vi "Main Tclk.vi"() -> ()   [LabVIEW 2018] (continued)
                        n671 = local read "Email recipents file"() -> (w5881:path)
                        n672 = Open/Create/Replace File(file path (use dialog)=w5881, operation (0:open)=T49."replace or create") -> (refnum out=w5882:refnum<file>, error out=w5883:errorcluster)  [unwired: 4 in, 1 out]
                        n673 = Write to Text File(file (use dialog)=w5882, text=w5884, error in=w5883) -> (refnum out=w5885:refnum<file>, error out=w5886:errorcluster)  [unwired: 1 in, 1 out]
                        n674 = Close File(refnum=w5885, error in=w5886) -> ()  [unwired: 2 out]
                      }
                      frame #4 {
                        n675 = local read "Hardware Configuration"() -> (w5948:T25)
                        n676 = local read "SEM Scan Parameters"() -> (w5932:T26)
                        n677 = local read "SEM Options"() -> (w5949:T27)
                        n678 = local read "SEM Status"() -> (w5950:T12)
                        n679 = local read "X full scale (V)"() -> (w5951:sgl)
                        n680 = local read "Mid Mag SEM"() -> (w5947:T29)
                        n681 = local read "SEM Mid Mag Scan Parameters"() -> (w5946:T5)
                        n682 = Unbundle By Name(w5947) -> ("X size (um)"=w5943:sgl, "Y size (um)"=w5942:sgl, "X center (um)"=w5941:dbl, "Y center (um)"=w5940:dbl, "Mid mag scan rate (Hz)"=w5945:u32, "Pixel size (nm)"=w5944:sgl)
                        n683 = call "SEM Scan Parameter Coerce.vi"("X full scale (V)"=w5951, "AI upper limit"=50000000.0, "SEM Status"=w5950, "SEM Options"=w5949, "SEM Scan Parameters"=w5932, "Hardware Configuration"=w5948) -> ("Coerced SEM Scan Parameters"=w5952:T5, "SEM FOV"=w5931:dbl, "Detector number"=w5930:i16)  [unwired: 3 in]
                        n684 = local write "Detector number"(w5930) -> ()
                        n685 = local write "SEM FOV"(w5931) -> ()
                        n686 = Bundle By Name(cluster=w5946, "X size (um)"=w5943, "Y size (um)"=w5942, "X center (um)"=w5941, "Y center (um)"=w5940, "Scan rate (Hz)"=w5945, "Pixel size (nm)"=w5944, "X size auto"=TRUE) -> (w5939:T5)
                        n687 = call "SEM Scan Parameter Coerce.vi"("X full scale (V)"=w5951, "SEM Status"=w5950, "SEM Options"=w5949, "SEM Scan Parameters"=w5939, "Hardware Configuration"=w5948) -> ("Coerced SEM Scan Parameters"=w5953:T5)  [unwired: 4 in, 2 out]
                        n688 = Unbundle By Name(w5953) -> ("X size (um)"=w5938:sgl, "Y size (um)"=w5937:sgl, "X center (um)"=w5936:dbl, "Y center (um)"=w5935:dbl, "Scan rate (Hz)"=w5934:u32, "Pixel size (nm)"=w5933:sgl)
                        n689 = Bundle By Name(cluster=w5947, "X size (um)"=w5938, "Y size (um)"=w5937, "X center (um)"=w5936, "Y center (um)"=w5935, "Mid mag scan rate (Hz)"=w5934, "Pixel size (nm)"=w5933) -> (w5954:T29)
                        n690 = local write "SEM Scan Parameters"(w5952) -> ()
                        n691 = local write "SEM Mid Mag Scan Parameters"(w5953) -> ()
                        n692 = local write "Mid Mag SEM"(w5954) -> ()
                      }
                      frame #5 {
                        n693 = local read "Reheat from last"() -> (w5955:bool)
                        n694 = case shown="True" w5955 {
                          frame False {
                          }
                          frame True {
                            n695 = local read "SEM Scan Parameters"() -> (w5960:T26)
                            n696 = Unbundle By Name(w5960) -> ("X center (um)"=w5959:sgl, "Y center (um)"=w5958:sgl, "Y stig"=w5957:sgl[][])
                            n697 = local write "Pre-reheat X center (um)"(w5959) -> ()
                            n698 = local write "Pre-reheat Y center (um)"(w5958) -> ()
                            n699 = local write "Pre-reheat Y stig"(w5957) -> ()
                            n700 = local write "Status Tabs"(T11."Re-engage" ("Status Tabs")) -> ()
                          }
                        }
                      }
                    }
                  }
                }
              }
              frame #1 {
                n701 = local read "Machine Type"() -> (w5977:u8)
                n702 = local read "Milling para"() -> (w5975:T35)
                n703 = Unbundle By Name(w5975) -> ("Lines auto pause"=w5974:u16)
                n704 = case shown="2" w5977 {
                  tunnel: [w5986 w5994 w5998] -> w5978
                  frame 0, Default {
                    n705 = for {
                      N: 10 -> [_]
                      tunnel: [w5991] -> w5988 mode=indexing
                      n706 = shared-variable ".\\Zeiss Library.lvlib\\Logs"() -> (w5993:sgl[])  [unwired: 1 in, 1 out]
                      n707 = Wait Until Next ms Multiple(millisecond multiple=u32 10) -> ()  [unwired: 1 out]
                      n708 = Index Array(array=w5993, index=0) -> (element=w5991:sgl)
                    }
                    n709 = call-poly <vilib>:"Basic Averaged DC-RMS.vi"("signal in"=w5988) -> ("DC value"=w5987:dbl)  [unwired: 7 in, 3 out]
                    n710 = To Single Precision Float(number=w5987) -> (single precision float=w5986:sgl)
                  }
                  frame 1 {
                    n711 = local read "Faraday Cup (nA)"() -> (w5994:sgl)
                  }
                  frame 2 {
                    n712 = local read "Api"() -> (w5997:refnum<k7>)
                    n713 = for {
                      N: 10 -> [_]
                      tunnel: [w6003] -> w6000 mode=indexing
                      n714 = shared-variable ".\\Zeiss Library.lvlib\\Logs"() -> (w6005:sgl[])  [unwired: 1 in, 1 out]
                      n715 = Wait Until Next ms Multiple(millisecond multiple=u32 10) -> ()  [unwired: 1 out]
                      n716 = Index Array(array=w6005, index=0) -> (element=w6003:sgl)
                    }
                    n717 = call "SmartSEM Remote API set float.vi"("vValue"=sgl 1.0, "lpszParam"="DP_PANEL_DISABLE", "ActiveX Container"=w5997) -> ()  [unwired: 7 in, 2 out]
                    n718 = call-poly <vilib>:"Basic Averaged DC-RMS.vi"("signal in"=w6000) -> ("DC value"=w5999:dbl)  [unwired: 7 in, 3 out]
                    n719 = To Single Precision Float(number=w5999) -> (single precision float=w5998:sgl)
                  }
                }
                "Faraday Cup before mill" <- w5978
                n720 = Equal?(x=w5974, y=u16 1) -> (x = y?=w5967:bool)
                n721 = case shown="True" w5967 {
                  tunnel: [0 w5980] -> w5966
                  frame False {
                  }
                  frame True {
                    n722 = local read "Continued fine milling frames"() -> (w5981:i32)
                    n723 = Increment(x=w5981) -> (x+1=w5980:i32)
                  }
                }
                n724 = local read "EHT off"() -> (w5970:bool)
                n725 = local read "Faraday Cup (nA)"() -> (w5972:sgl)
                n726 = local read "SEM Options"() -> (w5976:T27)
                n727 = Not(x=w5970) -> (.not. x?=w5969:bool)
                n728 = Unbundle By Name(w5976) -> ("Upload"=w5962:bool)
                n729 = Greater?(x=w5972, y=sgl 0.1) -> (0:w5968:bool)
                n730 = shared-variable ".\\Zeiss Library.lvlib\\Faraday Cup before mill"(w5978) -> ()  [unwired: 1 in, 1 out]
                n731 = local write "Continued fine milling frames"(w5966) -> ()
                n732 = Greater?(x=w5966, y=5) -> (0:w5964:bool)
                n733 = Compound Arithmetic op=AND(w5964, w5969, w5968) -> (w5963:bool)
                n734 = Or(x=w5963, y=w5962) -> (x .or. y?=w5961:bool)
                n735 = case shown="True" w5961 {
                  frame False {
                  }
                  frame True {
                    w5983 = TRUE ("Upload")
                    n736 = local read "Alert Settings"() -> (w5985:T36)
                    n737 = Bundle By Name(cluster=w5985, "3D imaging paused alarm"=w5983, "FIB emission warning"=w5983, "Specimen @ SEM alarm"=w5983, "FIB CL current alarm"=w5983, "Beam Dump 1 alarm"=w5983, "Milling Z voltage alarm"=w5983, "EHT off alarm"=w5983, "Image clipping alarm"=w5983, "Temperature alarm"=w5983, "SW error warning"=w5983, "Focus index warning"=w5983) -> (w5984:T36)
                    n738 = local write "Coarse milling"(FALSE ("Coarse milling")) -> ()
                    n739 = local write "Alert Settings"(w5984) -> ()
                  }
                }
              }
              frame #2 {
                w6007 = FALSE ("Rect Milling Line Paused")
                w6008 = TRUE ("Auto pause")
                n740 = local read "Milling para"() -> (w6006:T35)
                n741 = Bundle By Name(cluster=w6006, "Auto pause"=w6008) -> (w6009:T35)
                n742 = shared-variable "My Computer\\Zeiss Library.lvlib\\Milling Resume"(w6008) -> ()  [unwired: 1 in, 1 out]
                n743 = shared-variable "My Computer\\Zeiss Library.lvlib\\Milling Line Paused"(w6007) -> ()  [unwired: 1 in, 1 out]
                n744 = local write "Mill Stop"(w6007) -> ()
                n745 = local write "Milling para"(w6009) -> ()
              }
              frame #3 {
                n746 = local read "FIB slice #"() -> (w6011:u32)
                n747 = Equal To 0?(x=w6011) -> (x = 0?=w6010:bool)
                n748 = case shown="True" w6010 {
                  frame False {
                  }
                  frame True {
                    n749 = stacked-sequence {
                      frame #0 {
                        w6012 = u8 100 ("Restart flag")
                        w6028 = 0.0
                        w6039 = TRUE ("Temperature warning armed")
                        w6017 = u32[] [] ("Log time array")
                        w6015 = sgl[] []
                        n750 = local write "SW error warning armed"(w6039) -> ()
                        n751 = local write "Focus index warning armed"(w6039) -> ()
                        n752 = local write "Temperature warning armed"(w6039) -> ()
                        n753 = local write "Re-engage warning armed"(w6039) -> ()
                        n754 = shared-variable ".\\Zeiss Library.lvlib\\FIB PID reset"(w6039) -> ()  [unwired: 1 in, 1 out]
                        n755 = Get Date/Time In Seconds() -> (seconds since 1Jan1904=w6038:timestamp)
                        n756 = To Double Precision Float(number=w6038) -> (double precision float=w6033:dbl)
                        n757 = Bundle(w6028, w6028) -> (w6027:cluster{dbl, dbl})  [unwired: 1 in]
                        n758 = Add(x=w6033, y=86400.0 ("X Scale.Range:Maximum")) -> (x+y=w6035:dbl)
                        n759 = Initialize Array(w6027, 0) -> (w6030:cluster{dbl, dbl}[])
                        n760 = Add(x=w6033, y=0.0 ("X Scale.Range:Minimum")) -> (x+y=w6031:dbl)
                        n761 = Bundle By Name(cluster="Additional Info", "Restart flag"=w6012, "Stage move flag"=w6012) -> (w6013:cluster{"Restart flag":u8, "Stage move flag":u8})
                        n762 = local read "SEM Scan Parameters"() -> (w6021:T26)
                        n763 = property on="FIB HV DataLog" class="WFChart (strict)"("History Data"=w6030, "XScale.Offset"=w6033, "XScale.Minimum"=w6031, "XScale.Maximum"=w6035, "XScale.Increment"=14400.0 ("X Scale.Range:Increment"), "XScale.MinorInc"=3600.0 ("X Scale.Range:Minor Increment")) -> ()  [unwired: 2 in, 2 out]
                        n764 = local write "Additional Info"(w6013) -> ()
                        n765 = Unbundle By Name(w6021) -> ("Y tiles"=w6020:u8, "X tiles"=w6019:u8)
                        n766 = Initialize Array(FALSE ("run minimized? (F)"), w6020, w6019) -> (w6022:bool[][])
                        n767 = local read "3D FIB-SEM Files"() -> (w6025:path)
                        n768 = local write "AF Success tiled"(w6022) -> ()
                        n769 = local write "ASX Success tiled"(w6022) -> ()
                        n770 = local write "ASY Success tiled"(w6022) -> ()
                        n771 = local write "AAX Success tiled"(w6022) -> ()
                        n772 = local write "AAY Success tiled"(w6022) -> ()
                        n773 = local write "Auto re-engage"(FALSE ("Auto re-engage")) -> ()
                        n774 = call <vilib>:"System Exec.vi"("run minimized? (F)"=TRUE, "working directory"=w6025, "command line"="cmd /c del Primary_grid*.png pre*.png post*.png") -> ()  [unwired: 5 in, 4 out]
                        "Temp array" <- w6015
                        "Faraday Cup array" <- w6015
                        "Specimen I array" <- w6015
                        "Beam Dump 1 array" <- w6015
                        "Log time array" <- w6017
                        "Delta X array" <- w6015
                        "Delta Y array" <- w6015
                        "Delta image array" <- w6015
                        "Focus index array" <- w6015
                        "Delta X sum array" <- w6015
                        "Delta Y sum array" <- w6015
                        "SEM Specimen I array" <- w6015
                        "Milling Z voltage array" <- w6015
                        "Delta Z array" <- w6015
                        "Beam Dump 2 array" <- w6015
                        "Milling I array" <- w6015
                        "Temp low limit array" <- w6015
                        "Temp high limit array" <- w6015
                        "SEM Specimen I low limit array" <- w6015
                        "SEM Specimen I high limit array" <- w6015
                        "FI low limit array" <- w6015
                        "Specimen I low limit array" <- w6015
                        "Specimen I high limit array" <- w6015
                        "Faraday Cup low limit array" <- w6015
                        "Faraday Cup high limit array" <- w6015
                        "Cycle time array" <- w6017
                        "Cycle time est offset array" <- i16[] [] ("Log time array")
                        "BD1 low limit array" <- w6015
                        "BD1 high limit array" <- w6015
                        "BD2 low limit array" <- w6015
                        "BD2 high limit array" <- w6015
                        "Milling I low limit array" <- w6015
                        "Milling I high limit array" <- w6015
                        "FI low warning limit array" <- w6015
                        "FI high warning limit array" <- w6015
                        "FI low stop limit array" <- w6015
                        "FI high stop limit array" <- w6015
                        "Delta X stop limit array" <- w6015
                        "Delta Y stop limit array" <- w6015
                        "FI array for stop limit" <- w6015
                        "Delta X array for stop limit" <- w6015
                        "Delta Y array for stop limit" <- w6015
                        "FRC array" <- w6015
                      }
                      frame #1 {
                        n775 = local read "SEM Scan Parameters"() -> (w6066:T26)
                        n776 = Unbundle By Name(w6066) -> ("WD (mm)"=w6065:sgl[][], "X stig"=w6062:sgl[][], "Y stig"=w6059:sgl[][], "X aln"=w6058:sgl[][], "Y aln"=w6056:sgl[][], "dX (um)"=w6054:sgl[], "dY (um)"=w6049:sgl[], "Y tiles"=w6052:u8, "X tiles"=w6050:u8)
                        n777 = local read "WD Stig Aln tile offsets"() -> (w6068:T3)
                        n778 = Build Array(w6052, w6050) -> (w6055:u8[])
                        n779 = Array Size(array=w6065) -> (size(s)=w6064:i32[])
                        n780 = Array Size(array=w6062) -> (size(s)=w6063:i32[])
                        n781 = Array Size(array=w6059) -> (size(s)=w6060:i32[])
                        n782 = Array Size(array=w6058) -> (size(s)=w6061:i32[])
                        n783 = Array Size(array=w6056) -> (size(s)=w6057:i32[])
                        n784 = Array Size(array=w6054) -> (size(s)=w6053:i32)
                        n785 = Array Size(array=w6049) -> (size(s)=w6051:i32)
                        n786 = Equal?(x=w6064, y=w6055) -> (x = y?=w6047:bool[])
                        n787 = Equal?(x=w6063, y=w6055) -> (x = y?=w6046:bool[])
                        n788 = Equal?(x=w6060, y=w6055) -> (x = y?=w6044:bool[])
                        n789 = Equal?(x=w6061, y=w6055) -> (x = y?=w6043:bool[])
                        n790 = Equal?(x=w6057, y=w6055) -> (x = y?=w6042:bool[])
                        n791 = Equal?(x=w6053, y=w6052) -> (x = y?=w6041:bool)
                        n792 = Equal?(x=w6051, y=w6050) -> (x = y?=w6040:bool)
                        n793 = Build Array (concatenate)(w6047, w6046, w6044, w6043, w6042, w6041, w6040) -> (w6045:bool[])
                        n794 = And Array Elements(Boolean array=w6045) -> (logical AND=w6048:bool)
                        n795 = case shown="True" w6048 {
                          tunnel: [w6069 w6097] -> w6067
                          tunnel: w6066 -> [w6071 w6091]
                          tunnel: w6068 -> [w6070 w6078]
                          frame False {
                            w6073 = sgl 0.0 ("element")
                            n796 = Unbundle By Name(w6071) -> ("Y tiles"=w6075:u8, "X tiles"=w6077:u8)
                            n797 = Initialize Array(w6073, w6075, w6077) -> (w6076:sgl[][])
                            n798 = Initialize Array(w6073, w6075) -> (w6074:sgl[])
                            n799 = Initialize Array(w6073, w6077) -> (w6072:sgl[])
                            n800 = Bundle By Name(cluster=w6070, "dWD"=w6076, "dX stig"=w6076, "dY stig"=w6076, "dX aln"=w6076, "dY aln"=w6076, "dX (um)"=w6074, "dY (um)"=w6072) -> (w6069:T3)
                          }
                          frame True {
                            n801 = Unbundle By Name(w6091) -> ("WD (mm)"=w6087:sgl[][], "X stig"=w6085:sgl[][], "Y stig"=w6082:sgl[][], "X aln"=w6081:sgl[][], "Y aln"=w6079:sgl[][], "dX (um)"=w6098:sgl[], "dY (um)"=w6103:sgl[], "Y tiles"=w6090:u8, "X tiles"=w6089:u8)
                            n802 = expression code="(x-1)/2"(w6090) -> (w6101:u8)
                            n803 = expression code="(x-1)/2"(w6089) -> (w6104:u8)
                            n804 = Index Array(array=w6087, index (row)=w6101, index (col)=w6104) -> (element=w6088:sgl)
                            n805 = Index Array(array=w6085, index (row)=w6101, index (col)=w6104) -> (element=w6086:sgl)
                            n806 = Index Array(array=w6082, index (row)=w6101, index (col)=w6104) -> (element=w6083:sgl)
                            n807 = Index Array(array=w6081, index (row)=w6101, index (col)=w6104) -> (element=w6084:sgl)
                            n808 = Index Array(array=w6079, index (row)=w6101, index (col)=w6104) -> (element=w6080:sgl)
                            n809 = Index Array(array=w6098, index=w6101) -> (element=w6099:sgl)
                            n810 = Index Array(array=w6103, index=w6104) -> (element=w6102:sgl)
                            n811 = Subtract(x=w6087, y=w6088) -> (x-y=w6092:sgl[][])
                            n812 = Subtract(x=w6085, y=w6086) -> (x-y=w6093:sgl[][])
                            n813 = Subtract(x=w6082, y=w6083) -> (x-y=w6094:sgl[][])
                            n814 = Subtract(x=w6081, y=w6084) -> (x-y=w6095:sgl[][])
                            n815 = Subtract(x=w6079, y=w6080) -> (x-y=w6096:sgl[][])
                            n816 = Subtract(x=w6098, y=w6099) -> (x-y=w6100:sgl[])
                            n817 = Subtract(x=w6103, y=w6102) -> (x-y=w6105:sgl[])
                            n818 = Bundle By Name(cluster=w6078, "dWD"=w6092, "dX stig"=w6093, "dY stig"=w6094, "dX aln"=w6095, "dY aln"=w6096, "dX (um)"=w6100, "dY (um)"=w6105) -> (w6097:T3)
                          }
                        }
                        n819 = local write "WD Stig Aln tile offsets"(w6067) -> ()
                      }
                    }
                  }
                }
              }
              frame #4 {
                n820 = Unbundle By Name("Low Mag SEM") -> ("Low mag scan"=w6108:bool)
                n821 = Unbundle By Name("Mid Mag SEM") -> ("Mid mag scan"=w6109:bool)
                n822 = case shown="True" w6108 {
                  tunnel: "Low Mag SEM" -> [_ w6132]
                  frame False {
                  }
                  frame True {
                    w6128 = sgl[] [0.0] ("dX (um)")
                    w6129 = u8 1 ("X tiles")
                    w6133 = 0.0 ("X center")
                    n823 = Unbundle By Name(w6132) -> ("Low mag scan FOV (micron)"=w6130:dbl, "Low mag scan rate (Hz)"=w6142:u32)
                    n824 = local read "SEM Scan Parameters"() -> (w6135:T26)
                    n825 = Unbundle By Name(w6135) -> ("Scan rate (Hz)"=w6137:u32, "Oversampling"=w6136:u32)
                    n826 = expression code="x*1000"(w6130) -> (w6143:dbl)
                    n827 = Multiply(x=w6137, y=w6136) -> (x*y=w6138:u32)
                    n828 = Divide(x=w6138, y=w6142) -> (x/y=w6139:dbl)
                    n829 = Divide(x=w6143, y=u32 512 ("X resolution")) -> (x/y=w6141:dbl)
                    n830 = Bundle By Name(cluster=w6135, "X size (um)"=w6130, "Y size (um)"=w6130, "X center (um)"=w6133, "Y center (um)"=w6133, "X size (V)"=20.0, "Scan rate (Hz)"=w6142, "Oversampling"=w6139, "X tiles"=w6129, "Y tiles"=w6129, "Frames"=w6129, "dX (um)"=w6128, "dY (um)"=w6128, "Pixel size (nm)"=w6141) -> (→"SEM Low Mag Scan Parameters":T26)
                  }
                }
                n831 = case shown="True" w6109 {
                  tunnel: "Mid Mag SEM" -> [_ w6116]
                  frame False {
                  }
                  frame True {
                    w6110 = sgl[] [0.0] ("dX (um)")
                    w6111 = u8 1 ("X tiles")
                    n832 = local read "SEM Scan Parameters"() -> (w6117:T26)
                    n833 = Unbundle By Name(w6116) -> ("X size (um)"=w6123:sgl, "Y size (um)"=w6124:sgl, "X center (um)"=w6125:dbl, "Y center (um)"=w6126:dbl, "Mid mag scan rate (Hz)"=w6122:u32, "Pixel size (nm)"=w6127:sgl)
                    n834 = local read "SEM Mid Mag Scan Parameters"() -> (w6114:T5)
                    n835 = Unbundle By Name(w6117) -> ("Scan rate (Hz)"=w6119:u32, "Oversampling"=w6118:u32)
                    n836 = Unbundle By Name(w6114) -> ("X size (V)"=w6113:dbl)
                    n837 = Multiply(x=w6119, y=w6118) -> (x*y=w6120:u32)
                    n838 = Divide(x=w6120, y=w6122) -> (x/y=w6121:dbl)
                    n839 = Bundle By Name(cluster=w6117, "X size (um)"=w6123, "Y size (um)"=w6124, "X center (um)"=w6125, "Y center (um)"=w6126, "Oversampling auto"=TRUE ("X size auto"), "Scan rate (Hz)"=w6122, "Oversampling"=w6121, "Pixel size (nm)"=w6127, "X size (V)"=w6113, "X tiles"=w6111, "Y tiles"=w6111, "Frames"=w6111, "dX (um)"=w6110, "dY (um)"=w6110) -> (→"SEM Mid Mag Scan Parameters":T26)
                  }
                }
              }
              frame #5 {
                w6144 = TRUE ("Mill")
                n840 = local write "Mill"(w6144) -> ()
                n841 = local write "Run once"(w6144) -> ()
                n842 = Wait (ms)(milliseconds to wait=u32 200) -> ()  [unwired: 1 out]
              }
              frame #6 {
                n843 = local read "Fail #"() -> (w6147:u8)
                n844 = shared-variable ".\\Zeiss Library.lvlib\\Milling Z Voltage"() -> (w6149:sgl)  [unwired: 1 in, 1 out]
                n845 = local read "FIB Options"() -> (w6158:T33)
                n846 = local read "FIB Scan Parameters"() -> (w6156:T32)
                n847 = local read "Milling para"() -> (w6155:T35)
                n848 = Greater Than 0?(x=w6147) -> (x > 0?=w6146:bool)
                n849 = Unbundle By Name(w6158) -> ("Flip z"=w6163:bool)
                n850 = Unbundle By Name(w6155) -> ("FIB FOV (um)"=w6162:sgl)
                n851 = Unbundle By Name(w6155) -> ("X size (um)"=w6153:sgl, "Line milling time (s)"=w6151:sgl, "Lines auto pause"=w6150:u16)
                n852 = local write "SEM shutter failed active"(w6146) -> ()
                n853 = Unbundle By Name(w6156) -> ("Z size (V)"=w6157:dbl)
                n854 = Negate(x=w6149) -> (-x=w6159:sgl)
                n855 = Select(t=w6159, s=w6163, f=w6149) -> (s? t:f=w6160:sgl)
                n856 = Divide(x=w6160, y=w6157) -> (x/y=w6161:dbl)
                n857 = Multiply(x=w6161, y=w6162) -> (x*y=w6148:dbl)
                n858 = call "Milling parameter to trapezoidal shape.vi"("Y location (um)"=w6148, "Milling para"=w6155) -> ("X size (um) @ Y"=w6154:dbl)  [unwired: 5 in, 4 out]
                n859 = Divide(x=w6154, y=w6153) -> (x/y=w6152:dbl)
                n860 = Compound Arithmetic op=MULTIPLY(w6152, w6151, w6150) -> (w6164:dbl)
                n861 = local write "Milling time (s)"(w6164) -> ()
              }
              frame #7 {
                n862 = while {
                  tunnel: [w6195] -> w6166
                  tunnel: [w6189] -> w6167
                  i -> [w6171]
                  stop <- w6196 stop-if-true
                  n863 = Get Date/Time In Seconds() -> (seconds since 1Jan1904=w6185:timestamp)
                  n864 = local read "Re-engage time"() -> (w6179:timestamp)
                  n865 = local read "Milling para"() -> (w6182:T35)
                  n866 = local read "Pre-reheat FIB PID target"() -> (w6178:sgl)
                  n867 = local read "Run once"() -> (w6176:bool)
                  n868 = shared-variable "My Computer\\Zeiss Library.lvlib\\Milling Line Paused"() -> (w6190:bool)  [unwired: 1 in, 1 out]
                  n869 = local read "Mill Manual Pause"() -> (w6194:bool)
                  n870 = local read "Machine Type"() -> (w6172:u8)
                  n871 = local read "Auto reheat running"() -> (w6170:bool)
                  n872 = local read "Reheat Output"() -> (w6188:T21)
                  n873 = local read "Stop"() -> (w6195:bool)
                  n874 = Wait Until Next ms Multiple(millisecond multiple=u32 100 ("milliseconds to wait")) -> ()  [unwired: 1 out]
                  n875 = Unbundle By Name(w6182) -> ("FIB PID on"=w6180:bool)
                  n876 = local read "FIB"() -> (w6192:bool)
                  n877 = Subtract(x=w6185, y=w6179) -> (x-y=w6184:dbl)
                  n878 = Unbundle By Name(w6188) -> ("Reheat Success"=w6187:bool)
                  n879 = Not Equal To 0?(x=w6178) -> (x != 0?=w6175:bool)
                  n880 = Not(x=w6192) -> (.not. x?=w6189:bool)
                  n881 = expression code="x/60"(w6184) -> (w6177:dbl)
                  n882 = case shown="False" w6194 {
                    tunnel: T44."Disabled and Grayed Out" ("Disabled") -> [w6299 _]
                    tunnel: T44."Enabled" ("Disabled") -> [_ w6317]
                    tunnel: w6172 -> [w6298 w6316]
                    tunnel: w6171 -> [w6297 w6315]
                    tunnel: w6170 -> [_ w6314]
                    frame False {
                      n883 = stacked-sequence {
                        tunnel: w6299 -> [_ w6304 w6305 _ _]
                        tunnel: w6298 -> [_ _ _ w6306 w6310]
                        tunnel: w6297 -> [w6301 _ _ _ _]
                        frame #0 {
                          n884 = Equal To 0?(x=w6301) -> (x = 0?=w6300:bool)
                          n885 = case shown="True" w6300 {
                            frame False {
                            }
                            frame True {
                              n886 = local write "Start Current DataLog"(FALSE ("Start Current DataLog")) -> ()
                              n887 = local write "Status message"("FIB milling ..." ("Status message")) -> ()
                            }
                          }
                        }
                        frame #1 {
                          n888 = property on="Scan x1" class="Bool (strict)"("DisabledEnum"=w6304) -> ()  [unwired: 2 in, 2 out]
                          n889 = property on="Scan xn" class="Bool (strict)"("DisabledEnum"=w6304) -> ()  [unwired: 2 in, 2 out]
                          n890 = property on="Pre image" class="Bool (strict)"("DisabledEnum"=w6304) -> ()  [unwired: 2 in, 2 out]
                          n891 = property on="Post image" class="Bool (strict)"("DisabledEnum"=w6304) -> ()  [unwired: 2 in, 2 out]
                          n892 = property on="Reset" class="Bool (strict)"("DisabledEnum"=w6304) -> ()  [unwired: 2 in, 2 out]
                          n893 = property on="Start Current DataLog" class="Bool (strict)"("DisabledEnum"=w6304) -> ()  [unwired: 2 in, 2 out]
                        }
                        frame #2 {
                          n894 = property on="FIB Imaging" class="Bool (strict)"("DisabledEnum"=w6305) -> ()  [unwired: 2 in, 2 out]
                          n895 = property on="FIB time lapse" class="Bool (strict)"("DisabledEnum"=w6305) -> ()  [unwired: 2 in, 2 out]
                        }
                        frame #3 {
                          n896 = case shown="2" w6306 {
                            frame 0, Default {
                            }
                            frame 2 {
                              n897 = local read "Api"() -> (w6309:refnum<k7>)
                              n898 = call "SmartSEM Remote API set float.vi"("vValue"=sgl 1.0, "lpszParam"="DP_PANEL_DISABLE", "ActiveX Container"=w6309) -> ()  [unwired: 7 in, 2 out]
                            }
                          }
                        }
                        frame #4 {
                          n899 = case shown="2" w6310 {
                            frame 0, Default {
                            }
                            frame 2 {
                              n900 = local read "Api"() -> (w6313:refnum<k7>)
                              n901 = call "SmartSEM Remote API set float.vi"("vValue"=sgl 1.0, "lpszParam"="DP_JOYSTICK_DISABLE", "ActiveX Container"=w6313) -> ()  [unwired: 7 in, 2 out]
                            }
                          }
                        }
                      }
                    }
                    frame True {
                      n902 = stacked-sequence {
                        tunnel: w6317 -> [_ w6324 w6325 _ _ _]
                        tunnel: w6316 -> [_ _ _ w6326 w6330 _]
                        tunnel: w6315 -> [w6322 _ _ _ _ _]
                        tunnel: w6314 -> [w6321 _ _ _ _ _]
                        frame #0 {
                          n903 = Equal To 0?(x=w6322) -> (x = 0?=w6320:bool)
                          n904 = Not(x=w6321) -> (.not. x?=w6319:bool)
                          n905 = Compound Arithmetic op=AND(w6320, w6319) -> (w6318:bool)
                          n906 = case shown="True" w6318 {
                            frame False {
                            }
                            frame True {
                              n907 = local write "Status message"("Milling paused" ("Status message")) -> ()
                            }
                          }
                        }
                        frame #1 {
                          n908 = property on="Scan x1" class="Bool (strict)"("DisabledEnum"=w6324) -> ()  [unwired: 2 in, 2 out]
                          n909 = property on="Scan xn" class="Bool (strict)"("DisabledEnum"=w6324) -> ()  [unwired: 2 in, 2 out]
                          n910 = property on="Pre image" class="Bool (strict)"("DisabledEnum"=w6324) -> ()  [unwired: 2 in, 2 out]
                          n911 = property on="Post image" class="Bool (strict)"("DisabledEnum"=w6324) -> ()  [unwired: 2 in, 2 out]
                          n912 = property on="Reset" class="Bool (strict)"("DisabledEnum"=w6324) -> ()  [unwired: 2 in, 2 out]
                          n913 = property on="Start Current DataLog" class="Bool (strict)"("DisabledEnum"=w6324) -> ()  [unwired: 2 in, 2 out]
                        }
                        frame #2 {
                          n914 = property on="FIB time lapse" class="Bool (strict)"("DisabledEnum"=w6325) -> ()  [unwired: 2 in, 2 out]
                          n915 = property on="Pause for reheat" class="Bool (strict)"("DisabledEnum"=w6325) -> ()  [unwired: 2 in, 2 out]
                        }
                        frame #3 {
                          n916 = case shown="2" w6326 {
                            frame 0, Default {
                            }
                            frame 2 {
                              n917 = local read "Api"() -> (w6329:refnum<k7>)
                              n918 = call "SmartSEM Remote API set float.vi"("vValue"=sgl 0.0, "lpszParam"="DP_PANEL_DISABLE", "ActiveX Container"=w6329) -> ()  [unwired: 7 in, 2 out]
                            }
                          }
                        }
                        frame #4 {
                          n919 = case shown="2" w6330 {
                            frame 0, Default {
                            }
                            frame 2 {
                              n920 = local read "Api"() -> (w6333:refnum<k7>)
                              n921 = call "SmartSEM Remote API set float.vi"("vValue"=sgl 0.0, "lpszParam"="DP_JOYSTICK_DISABLE", "ActiveX Container"=w6333) -> ()  [unwired: 7 in, 2 out]
                            }
                          }
                        }
                        frame #5 {
                          n922 = local read "FIB HW Config"() -> (w6335:T23)
                          n923 = local read "Api"() -> (w6334:refnum<k7>)
                          n924 = Unbundle By Name(w6335) -> ("Beam blank"=w6336:tag)
                          n925 = call "FIB beam blank.vi"("ActiveX Container"=w6334, "Beam blanked"=TRUE, "lines"=w6336) -> ()  [unwired: 2 in, 1 out]
                        }
                      }
                    }
                  }
                  n926 = Subtract(x="Transition time (min)", y=w6177) -> (x-y=w6173:dbl)
                  n927 = Greater Than 0?(x=w6173) -> (x > 0?=w6174:bool)
                  n928 = Compound Arithmetic op=AND(w6174, w6180, w6175, w6176) -> (w6181:bool)
                  n929 = Compound Arithmetic op=AND(w6170, w6187) -> (w6186:bool)
                  n930 = case shown="True" w6181 {
                    tunnel: w6177 -> [_ w6223]
                    tunnel: "Transition time (min)" -> [_ w6222]
                    tunnel: w6182 -> [w6205 w6212]
                    tunnel: w6178 -> [w6202 w6211]
                    tunnel: w6175 -> [w6201 _]
                    tunnel: w6173 -> [w6200 _]
                    frame False {
                      n931 = Less Than 0?(x=w6200) -> (x < 0?=w6198:bool)
                      n932 = local read "PID recovered"() -> (w6203:bool)
                      n933 = Not(x=w6203) -> (.not. x?=w6199:bool)
                      n934 = Compound Arithmetic op=AND(w6199, w6198, w6201) -> (w6204:bool)
                      n935 = case shown="True" w6204 {
                        tunnel: w6205 -> [_ w6208]
                        tunnel: w6202 -> [_ w6207]
                        frame False {
                        }
                        frame True {
                          n936 = Bundle By Name(cluster=w6208, "FIB PID target"=w6207) -> (w6209:T35)
                          n937 = local write "Milling para"(w6209) -> ()
                          "PID recovered" <- TRUE
                        }
                      }
                    }
                    frame True {
                      w6210 = FALSE
                      n938 = Divide(x=w6223, y=w6222) -> (x/y=w6221:dbl)
                      n939 = expression code="x/100"("PID Target (%)") -> (w6216:sgl)
                      n940 = local write "PID recovered"(w6210) -> ()
                      n941 = Subtract(x=sgl 1.0, y=w6216) -> (x-y=w6217:sgl)
                      n942 = Multiply(x=w6221, y=w6217) -> (x*y=w6220:dbl)
                      n943 = Add(x=w6220, y=w6216) -> (x+y=w6218:dbl)
                      n944 = Multiply(x=w6218, y=w6211) -> (x*y=w6214:dbl)
                      n945 = Bundle By Name(cluster=w6212, "FIB PID target"=w6214) -> (w6213:T35)
                      n946 = local write "Milling para"(w6213) -> ()
                      "Run once" <- w6210
                    }
                  }
                  n947 = case shown="True" w6186 {
                    frame False {
                    }
                    frame True {
                      n948 = stacked-sequence {
                        seq-local: [_ w6225 _] -> [_ _ w6260]
                        frame #0 {
                          n949 = Wait (ms)(milliseconds to wait=u32 10000) -> ()  [unwired: 1 out]
                        }
                        frame #1 {
                          n950 = local read "Machine Type"() -> (w6226:u8)
                          n951 = case shown="2" w6226 {
                            tunnel: [w6227 w6235] -> w6225
                            frame 0, Default {
                              n952 = local read "HV Data Output"() -> (w6231:T18)
                              n953 = local read "Reheat Parameters"() -> (w6232:T1)
                              n954 = Unbundle By Name(w6231) -> ("Emission (uA)"=w6233:sgl)
                              n955 = Unbundle By Name(w6232) -> ("Emission (uA)"=w6234:sgl)
                              n956 = Subtract(x=w6233, y=w6234) -> (x-y=w6228:sgl)
                              n957 = Absolute Value(x=w6228) -> (abs(x)=w6229:sgl)
                              n958 = Greater?(x=0.1 ("y"), y=w6229) -> (0:w6227:bool)
                            }
                            frame 2 {
                              n959 = stacked-sequence {
                                tunnel: [_ w6259] -> w6235
                                frame #0 {
                                n960 = local read "FIB HV target matched"() -> (w6237:bool)
                                n961 = And(x="FIB probe auto min", y=w6237) -> (x .and. y?=w6238:bool)
                                n962 = case shown="True" w6238 {
                                frame False {
                                }
                                frame True {
                                n963 = local read "Api"() -> (w6242:refnum<k7>)
                                n964 = local read "FIB Milling Probe"() -> (w6240:string)
                                n965 = call "SmartSEM Remote API goto min or max FIB probe current.vi"("Min or Max"="Min", "FIB Probe"=w6240, "ActiveX Container"=w6242) -> ("Goto probe"=w6241:string)  [unwired: 7 in, 1 out]
                                n966 = local write "FIB Milling Probe"(w6241) -> ()
                                }
                                }
                                }
                                frame #1 {
                                n967 = local read "Api"() -> (w6243:refnum<k7>)
                                n968 = local read "FIB Parameters"() -> (w6258:T19)
                                n969 = call "SmartSEM Remote API FIB Faraday cup.vi"("ActiveX Container"=w6243) -> ("FIB Faraday Cup (nA)"=w6256:sgl)  [unwired: 8 in, 2 out]
                                n970 = call "SmartSEM Remote API get FIB HV data.vi"("ActiveX Container"=w6243) -> ("Capella HV Data Output"=w6245:T17)  [unwired: 7 in, 3 out]
                                n971 = Unbundle By Name(w6258) -> ("FIB probe current"=w6257:sgl)
                                n972 = Unbundle By Name(w6245) -> ("Emission Target (uA)"=w6247:sgl, "Emission Actual (uA)"=w6246:sgl)
                                n973 = local read "FIB HV target matched"() -> (w6251:bool)
                                n974 = Divide(x=w6256, y=w6257) -> (x/y=w6255:sgl)
                                n975 = Subtract(x=w6247, y=w6246) -> (x-y=w6250:sgl)
                                n976 = Absolute Value(x=w6250) -> (abs(x)=w6249:sgl)
                                n977 = In Range and Coerce(upper limit=sgl 1.5 ("y"), x=w6255, lower limit=sgl 0.8 ("y")) -> (In Range?=w6252:bool)  [unwired: 1 out]
                                n978 = Less?(x=w6249, y=sgl 0.1) -> (x < y?=w6244:bool)
                                n979 = Compound Arithmetic op=AND(w6251, w6252, w6244) -> (w6259:bool)
                                }
                              }
                            }
                          }
                        }
                        frame #2 {
                          n980 = case shown="True" w6260 {
                            frame False {
                            }
                            frame True {
                              n981 = stacked-sequence {
                                frame #0 {
                                w6266 = dbl[] [] ("Re-engage Delta X array")
                                w6267 = 0.0 ("Re-engage X shift")
                                n982 = local write "Re-engage X shift (um)"(w6267) -> ()
                                n983 = local write "Re-engage Y shift (um)"(w6267) -> ()
                                n984 = local write "Re-engage Delta X array"(w6266) -> ()
                                n985 = local write "Re-engage Delta Y array"(w6266) -> ()
                                n986 = local write "Re-engage X shift array"(w6266) -> ()
                                n987 = local write "Re-engage Y shift array"(w6266) -> ()
                                n988 = local read "Last milling snapshot"() -> (w6264:path)
                                n989 = call-poly <vilib>:"Read From XML File.vi"("XML File Path"=w6264) -> ("XML Elements"=w6265:string)  [unwired: 8 in, 2 out]
                                n990 = Unflatten From XML(xml string=w6265, type=T46 {"Timestamp"=timestamp(0 s since 1904-01-01), "Milling Z voltage"=0.0, "FIB slice #"=0, "Pause for reheat"=FALSE, "Last good FI"=0.0, "Focus index"=0.0, "SEM max FOV"=0.0, "Remaining X shift frames"=0, "Remaining Y shift frames"=0} ("output cluster")) -> (value=w6263:T46)  [unwired: 1 in, 1 out]
                                n991 = Unbundle By Name(w6263) -> ("Milling Z voltage"=w6262:sgl)
                                n992 = shared-variable ".\\Zeiss Library.lvlib\\Milling Z Voltage Last"(w6262) -> ()  [unwired: 1 in, 1 out]
                                }
                                frame #1 {
                                n993 = local read "Machine Type"() -> (w6269:u8)
                                n994 = case shown="2" w6269 {
                                tunnel: [w6270 w6278 w6279] -> w6268
                                frame 0, Default {
                                n995 = for {
                                N: 10 -> [_]
                                tunnel: [w6275] -> w6272 mode=indexing
                                n996 = shared-variable ".\\Zeiss Library.lvlib\\Logs"() -> (w6277:sgl[])  [unwired: 1 in, 1 out]
                                n997 = Index Array(array=w6277, index=0) -> (element=w6275:sgl)
                                n998 = Wait Until Next ms Multiple(millisecond multiple=u32 10) -> ()  [unwired: 1 out]
                                }
                                n999 = call-poly <vilib>:"Basic Averaged DC-RMS.vi"("signal in"=w6272) -> ("DC value"=w6271:dbl)  [unwired: 7 in, 3 out]
                                n1000 = To Single Precision Float(number=w6271) -> (single precision float=w6270:sgl)
                                }
                                frame 1 {
                                n1001 = local read "Faraday Cup (nA)"() -> (w6278:sgl)
                                }
                                frame 2 {
                                n1002 = for {
                                N: 10 -> [_]
                                tunnel: [w6284] -> w6281 mode=indexing
                                n1003 = shared-variable ".\\Zeiss Library.lvlib\\Logs"() -> (w6286:sgl[])  [unwired: 1 in, 1 out]
                                n1004 = Index Array(array=w6286, index=0) -> (element=w6284:sgl)
                                n1005 = Wait Until Next ms Multiple(millisecond multiple=u32 10) -> ()  [unwired: 1 out]
                                }
                                n1006 = call-poly <vilib>:"Basic Averaged DC-RMS.vi"("signal in"=w6281) -> ("DC value"=w6280:dbl)  [unwired: 7 in, 3 out]
                                n1007 = To Single Precision Float(number=w6280) -> (single precision float=w6279:sgl)
                                }
                                }
                                n1008 = shared-variable ".\\Zeiss Library.lvlib\\Faraday Cup before mill"(w6268) -> ()  [unwired: 1 in, 1 out]
                                n1009 = local write "Faraday Cup before mill"(w6268) -> ()
                                }
                                frame #2 {
                                w6290 = u8 0 ("Re-engage counts")
                                w6291 = FALSE ("Reheat")
                                n1010 = local write "Re-engage counts"(w6290) -> ()
                                n1011 = local write "Recovered counts"(w6290) -> ()
                                n1012 = local write "Last re-engage count"(w6290) -> ()
                                n1013 = local write "Pause for reheat"(w6291) -> ()
                                n1014 = local write "Mill Manual Pause"(w6291) -> ()
                                n1015 = local write "Reheat from last"(w6291) -> ()
                                n1016 = local read "Additional Info"() -> (w6289:cluster{"Restart flag":u8, "Stage move flag":u8})
                                n1017 = Bundle By Name(cluster=w6289, "Restart flag"=u8 1) -> (w6288:cluster{"Restart flag":u8, "Stage move flag":u8})
                                n1018 = local write "Additional Info"(w6288) -> ()
                                }
                                frame #3 {
                                w6293 = TRUE ("Reset WD")
                                n1019 = local read "Alert Settings"() -> (w6292:T36)
                                n1020 = local write "SW error warning armed"(w6293) -> ()
                                n1021 = local write "Auto re-engage"(w6293) -> ()
                                n1022 = local write "3D image paused armed"(w6293) -> ()
                                n1023 = local write "Temperature warning armed"(w6293) -> ()
                                n1024 = local write "Prior Alert Settings"(w6292) -> ()
                                }
                                frame #4 {
                                n1025 = Get Date/Time In Seconds() -> (seconds since 1Jan1904=w6294:timestamp)
                                n1026 = local write "Auto reheat running"(FALSE ("Auto reheat running")) -> ()
                                n1027 = local write "Re-engage time"(w6294) -> ()
                                n1028 = property on="Mill Manual Pause" class="Bool (strict)"("DisabledEnum"=T44."Enabled" ("Disabled")) -> ()  [unwired: 2 in, 2 out]
                                }
                              }
                            }
                          }
                        }
                      }
                    }
                  }
                  n1029 = Compound Arithmetic op=OR(w6190, w6189, w6195) -> (w6196:bool)
                }
                n1030 = case shown="True" w6166 {
                  frame False {
                  }
                  frame True {
                    w6169 = T44."Enabled" ("Disabled")
                    n1031 = property on="Scan x1" class="Bool (strict)"("DisabledEnum"=w6169) -> ()  [unwired: 2 in, 2 out]
                    n1032 = property on="Scan xn" class="Bool (strict)"("DisabledEnum"=w6169) -> ()  [unwired: 2 in, 2 out]
                    n1033 = property on="Start Current DataLog" class="Bool (strict)"("DisabledEnum"=w6169) -> ()  [unwired: 2 in, 2 out]
                    n1034 = property on="Pre image" class="Bool (strict)"("DisabledEnum"=w6169) -> ()  [unwired: 2 in, 2 out]
                    n1035 = property on="Post image" class="Bool (strict)"("DisabledEnum"=w6169) -> ()  [unwired: 2 in, 2 out]
                    n1036 = property on="Reset" class="Bool (strict)"("DisabledEnum"=w6169) -> ()  [unwired: 2 in, 2 out]
                    n1037 = property on="FIB time lapse" class="Bool (strict)"("DisabledEnum"=w6169) -> ()  [unwired: 2 in, 2 out]
                    n1038 = property on="FIB Imaging" class="Bool (strict)"("DisabledEnum"=w6169) -> ()  [unwired: 2 in, 2 out]
                  }
                }
                n1039 = Or(x=w6167, y=w6166) -> (x .or. y?=w6165:bool)
                n1040 = shared-variable "My Computer\\Zeiss Library.lvlib\\Milling Stop"(w6165) -> ()  [unwired: 1 in, 1 out]
                n1041 = shared-variable "My Computer\\Zeiss Library.lvlib\\Milling Resume"(FALSE ("Milling Resume")) -> ()  [unwired: 1 in, 1 out]
              }
              frame #8 {
